vi "high_pass_filter_3rd.vi"(7 "Input":dbl format="%.2f", 13 "Corner period":dbl(slide)=10.237739663395852 scale=1.0..1000.0) -> (8 "Output":dbl format="%.2f")   [LabVIEW 2016]
doc: "Use this VI to filter a signal using 3rd order high pass filter. The difference equation is \n[y(j)-3*y(j-1)+3*y(j-2)-y(j-3)] + 2*b*[y(j)-2*y(j-1)+y(j-2)] + 2*(b^2)*[y(j)-y(j-1)] + (b^3)*y(j) = [x(j)-3*x(j-1)+3*x(j-2)-x(j-3)].\n\nInputs:\nInput,\nCorner period.\nOutputs:\nOutput.\n\nMuhannad Alghamdi\nCSUSB Physics 350"
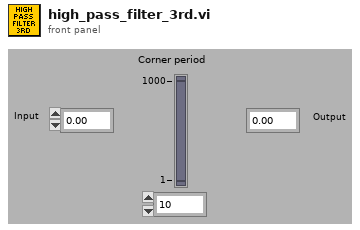
[diagram p1: front panel]
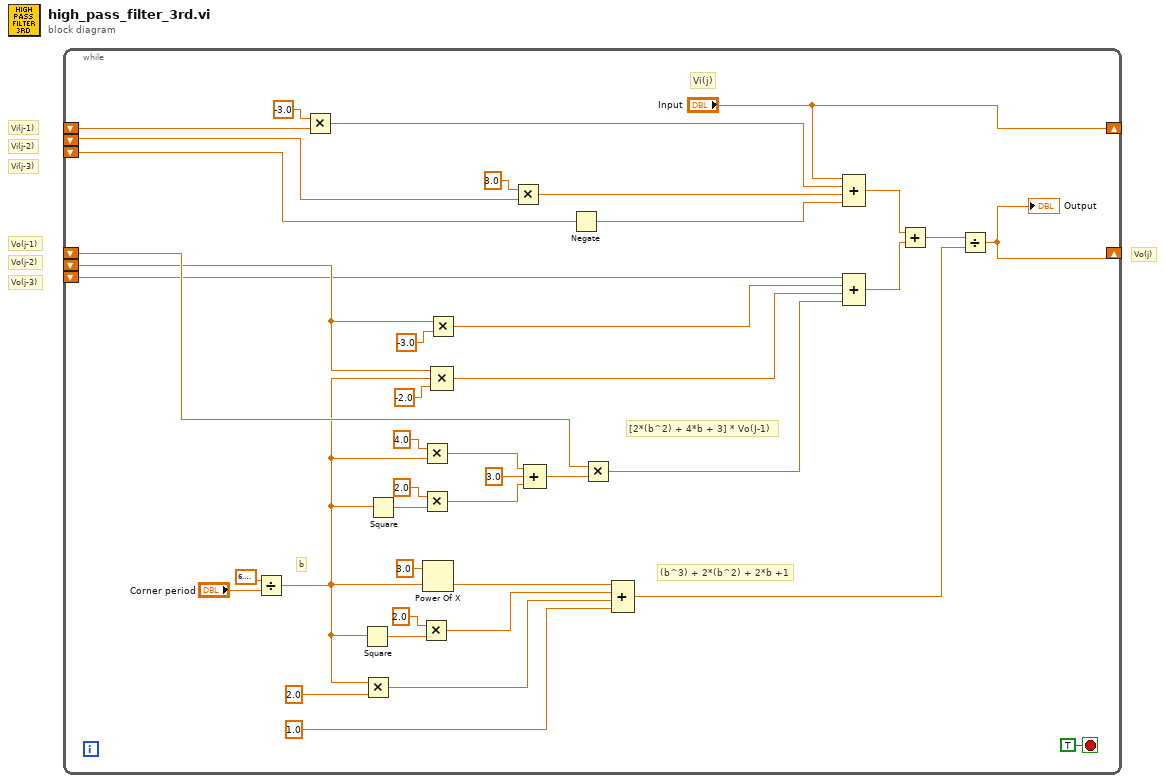
[diagram p0: block diagram]
diagram:
  # "Vi(j-3)"
  # "Vi(j-1)"
  # "Vi(j-2)"
  # "Vo(j-3)"
  # "Vo(j-1)"
  # "Vo(j-2)"
  # "Vo(j)"
  n1 = while {
    shift-left: _ -> [w21]
    shift-right: [w38] -> _
    shift-left: _ -> [w19]
    shift-left: _ -> [w15]
    shift-right: ["Input"] -> _
    shift-left: _ -> [w12]
    shift-left: _ -> [w7]
    shift-left: _ -> [w6]
    stop <- TRUE stop-if-true
    # "Vi(j)"
    # "[2*(b^2) + 4*b + 3] * Vo(J-1)"
    # "(b^3) + 2*(b^2) + 2*b +1"
    # "b"
    n2 = Divide(x=6.283185307179586, y="Corner period") -> (x/y=w14:dbl)
    n3 = Multiply(x=-3.0, y=w12) -> (x*y=w11:dbl)
    n4 = Square(x=w14) -> (x^2=w27:dbl)
    n5 = Multiply(x=w14, y=2.0 ("x")) -> (x*y=w36:dbl)
    n6 = Square(x=w14) -> (x^2=w33:dbl)
    n7 = Multiply(x=2.0, y=w27) -> (x*y=w25:dbl)
    n8 = Multiply(x=4.0, y=w14) -> (x*y=w31:dbl)
    n9 = Multiply(x=2.0, y=w33) -> (x*y=w30:dbl)
    n10 = Power Of X(1:w14, 2:3.0 ("y")) -> (0:w24:dbl)
    n11 = Multiply(x=w19, y=-3.0) -> (x*y=w16:dbl)
    n12 = Compound Arithmetic op=MULTIPLY(w19, w14, -2.0 ("value")) -> (w17:dbl)
    n13 = Multiply(x=3.0, y=w7) -> (x*y=w8:dbl)
    n14 = Compound Arithmetic op=ADD(w31, 3.0 ("value"), w30) -> (w22:dbl)
    n15 = Negate(x=w6) -> (-x=w5:dbl)
    n16 = Multiply(x=w21, y=w22) -> (x*y=w1:dbl)
    n17 = Compound Arithmetic op=ADD(w24, w25, w36, 1.0 ("value")) -> (w37:dbl)
    n18 = Compound Arithmetic op=ADD("Input", w11, w8, w5) -> (w4:dbl)
    n19 = Compound Arithmetic op=ADD(w15, w16, w17, w1) -> (w3:dbl)
    n20 = Add(x=w4, y=w3) -> (x+y=w2:dbl)
    n21 = Divide(x=w2, y=w37) -> (x/y=w38:dbl)
    "Output" <- w38
  }
